vi "initialize data references.vi"(8 "error in (no error)":errorcluster, 10 "Device Info in":T2 {"Outputs"."Output References"."Holding Registers" format="%.0x"; "Outputs"."Output References"."Coils" format="%.0x"; "Inputs"."Input References"."Input Registers" format="%.0x"; "Inputs"."Input References"."Discrete Inputs" format="%.0x"; "Interface Data"."Serial Settings"."parity (even)" items=["None", "Odd", "Even", "Mark", "Space"]; "Interface Data"."Serial Settings"."flow control (none)" items=["None", "XON/XOFF", "RTS/CTS", "XON/XOFF & RTS/CTS", "DTR/DSR", "XON/XOFF & DTR/DSR"]}, 11 "Item Ref in":T1 format="%.0x") -> (0 "error out":errorcluster, 2 "Device Info out":T2 {"Outputs"."Output References"."Holding Registers" format="%.0x"; "Outputs"."Output References"."Coils" format="%.0x"; "Inputs"."Input References"."Input Registers" format="%.0x"; "Inputs"."Input References"."Discrete Inputs" format="%.0x"; "Interface Data"."Serial Settings"."parity (even)" items=["None", "Odd", "Even", "Mark", "Space"]; "Interface Data"."Serial Settings"."flow control (none)" items=["None", "XON/XOFF", "RTS/CTS", "XON/XOFF & RTS/CTS", "DTR/DSR", "XON/XOFF & DTR/DSR"]}, 3 "Device Ref out":T1 format="%.0x")   [LabVIEW 2015]
uses:
  <vilib>/NI Veristand/Custom Device API/Data Access Type.ctl
  <vilib>/NI VeriStand/Custom Device API/Custom Device API.lvlib
  Modbus Master Engine.lvlib
  <vilib>/NI Veristand/Custom Device API/Custom Device Item Ref.ctl
  Shared/Controls/Interface Type.ctl
  System Explorer/Modbus Master System Explorer.lvlib
  Shared/Controls/Data Model/TCP Settings.ctl
  Shared/Modbus Master Shared.lvlib
  Shared/Controls/Data Model/Serial Settings.ctl
  Shared/Controls/Data Model/Input References.ctl
  System Explorer/SubVIs/Modbus Type.ctl
  Shared/Controls/Data Model/Channel.ctl
  Shared/Controls/Data Model/Input Channel Data.ctl
  Shared/Controls/Data Model/Inputs.ctl
  Shared/Controls/Data Model/Output Channel Data.ctl
  Shared/Controls/Data Model/Output References.ctl
  Shared/Controls/Data Model/Outputs.ctl
  Shared/Device Info.ctl
  Shared/Controls/Data Model/DataType.ctl
  Shared/Controls/Data Model/Mapping.ctl
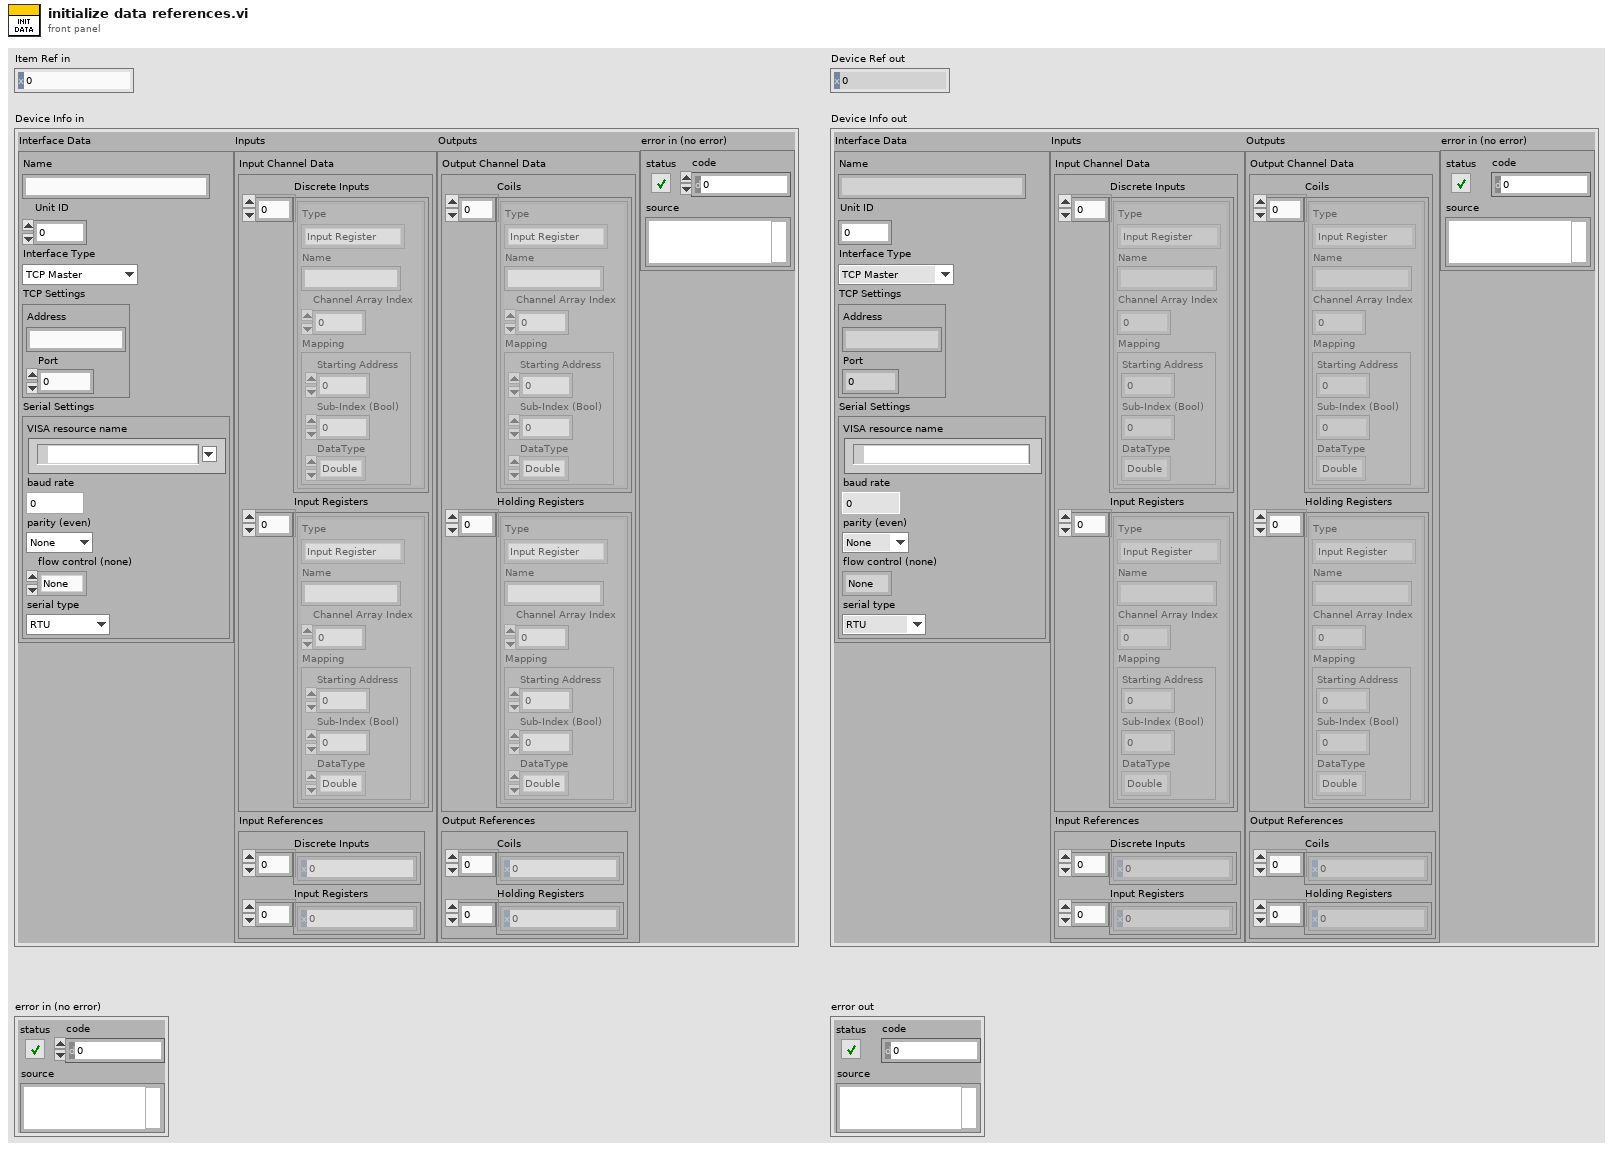
[diagram p1: front panel]
types:
  T1 = typedef "Custom Device API.lvlib/Custom Device Item Ref.ctl" = u64
  T2 = typedef "Modbus Master Shared.lvlib/Device Info.ctl" = cluster{"Interface Data":cluster{"Name":string, "Unit ID":u8, "Interface Type":T3, "TCP Settings":T4, "Serial Settings":T5}, "Inputs":T6, "Outputs":T13, "error in (no error)":errorcluster}
  T3 = typedef "Modbus Master System Explorer.lvlib/Interface Type.ctl" = enum16{"TCP Master", "Serial Master"}
  T4 = typedef "Modbus Master Shared.lvlib/TCP Settings.ctl" = cluster{"Address":string, "Port":u16}
  T5 = typedef "Modbus Master Shared.lvlib/Serial Settings.ctl" = cluster{"VISA resource name":refnum<visa-resource-name>, "baud rate":u32, "parity (even)":u16, "flow control (none)":u16, "serial type":enum16{"RTU", "ASCII"}}
  T6 = typedef "Modbus Master Shared.lvlib/Inputs.ctl" = cluster{"Input Channel Data":T7, "Input References":T12}
  T7 = typedef "Modbus Master Shared.lvlib/Input Channel Data.ctl" = cluster{"Discrete Inputs":T8[], "Input Registers":T8[]}
  T8 = typedef "Modbus Master Shared.lvlib/Channel.ctl" = cluster{"Type":T9, "Name":string, "Channel Array Index":i32, "Mapping":T10}
  T9 = typedef "Modbus Master Shared.lvlib/Modbus Type.ctl" = enum16{"Coil", "Discrete Input", "Holding Register", "Input Register"}
  T10 = typedef "Modbus Master Shared.lvlib/Mapping.ctl" = cluster{"Starting Address":u16, "Sub-Index (Bool)":u16, "DataType":T11}
  T11 = typedef "Modbus Master Shared.lvlib/DataType.ctl" = enum16{"Double", "Single", "I64", "I32", "I16", "I8", "U64", "U32", "U16", "U8", "Boolean", "String"}
  T12 = typedef "Modbus Master Shared.lvlib/Input References.ctl" = cluster{"Discrete Inputs":T1[], "Input Registers":T1[]}
  T13 = typedef "Modbus Master Shared.lvlib/Outputs.ctl" = cluster{"Output Channel Data":T14, "Output References":T15}
  T14 = typedef "Modbus Master Shared.lvlib/Output Channel Data.ctl" = cluster{"Coils":T8[], "Holding Registers":T8[]}
  T15 = typedef "Modbus Master Shared.lvlib/Output References.ctl" = cluster{"Coils":T1[], "Holding Registers":T1[]}
  T16 = typedef "Custom Device API.lvlib/Data Access Type.ctl" = enum16{"Read", "Write"}
  T17 = typedef "Custom Device API.lvlib/Data Reference.ctl" = i32
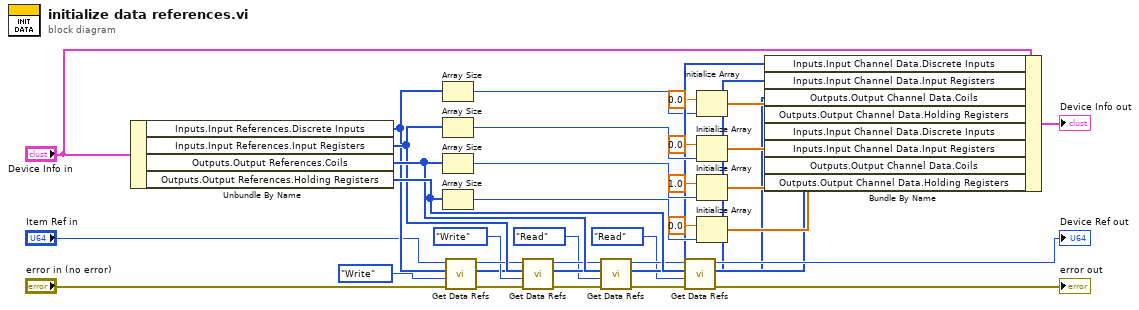
[diagram p0: block diagram]
diagram:
  n1 = Unbundle By Name("Device Info in") -> ("Inputs.Input References.Discrete Inputs"=w32:T1[], "Inputs.Input References.Input Registers"=w33:T1[], "Outputs.Output References.Coils"=w34:T1[], "Outputs.Output References.Holding Registers"=w35:T1[])
  n2 = Array Size(array=w32) -> (size(s)=w1:i32)
  n3 = Array Size(array=w33) -> (size(s)=w16:i32)
  n4 = Array Size(array=w34) -> (size(s)=w17:i32)
  n5 = Array Size(array=w35) -> (size(s)=w20:i32)
  n6 = call "Get Data Refs.vi"("error in (no error)"="error in (no error)", "Access"=Data_Access_Type."Write", "References"=w32, "Item Ref in"="Item Ref in") -> ("error out"=w29:errorcluster, "Data References"=w5:T17[], "Device Ref out"=w7:T1)  [unwired: 5 in]
  n7 = call "Get Data Refs.vi"("error in (no error)"=w29, "Access"=Data_Access_Type."Write", "References"=w33, "Item Ref in"=w7) -> ("error out"=w28:errorcluster, "Data References"=w12:T17[], "Device Ref out"=w10:T1)  [unwired: 5 in]
  n8 = call "Get Data Refs.vi"("error in (no error)"=w28, "Access"=Data_Access_Type."Read", "References"=w34, "Item Ref in"=w10) -> ("error out"=w27:errorcluster, "Data References"=w13:T17[], "Device Ref out"=w11:T1)  [unwired: 5 in]
  n9 = call "Get Data Refs.vi"("error in (no error)"=w27, "Access"=Data_Access_Type."Read", "References"=w35, "Item Ref in"=w11) -> ("error out"=→"error out":errorcluster, "Data References"=w14:T17[], "Device Ref out"=→"Device Ref out":T1)  [unwired: 5 in]
  n10 = Initialize Array(0.0 ("element"), w1) -> (w21:dbl[])
  n11 = Initialize Array(0.0 ("element"), w16) -> (w22:dbl[])
  n12 = Initialize Array(1.0 ("element"), w17) -> (w23:dbl[])
  n13 = Initialize Array(0.0 ("element"), w20) -> (w24:dbl[])
  n14 = Bundle By Name(cluster="Device Info in", "Inputs.Input Channel Data.Discrete Inputs"=w5, "Inputs.Input Channel Data.Input Registers"=w12, "Outputs.Output Channel Data.Coils"=w13, "Outputs.Output Channel Data.Holding Registers"=w14, "Inputs.Input Channel Data.Discrete Inputs"=w21, "Inputs.Input Channel Data.Input Registers"=w22, "Outputs.Output Channel Data.Coils"=w23, "Outputs.Output Channel Data.Holding Registers"=w24) -> (→"Device Info out":T2)
